vi "Image Display Loop.vi"(0 "fpga interface in":refnum<k20>, 1 "'stop' notifier":refnum<notifier>, 2 "rate references":T1(array[cluster]), 3 "Ctl Refnum":refnum<vi>, 5 "raw display notifier":refnum<notifier>, 7 "display references":refnum<vi>[](array[refnum]), 11 "error in (no error)":errorcluster) -> (15 "error out":errorcluster)   [LabVIEW 2025, in "GettingStarted_Common_148X_Host.lvlib"]
uses:
  GettingStarted_Common_148X_Host.lvlib
  <vilib>/vision/Image Controls.llb/IMAQ Image.ctl
  Types/Serial Channel Display Parameters.ctl
  Types/RAW Interpretation for Display.ctl
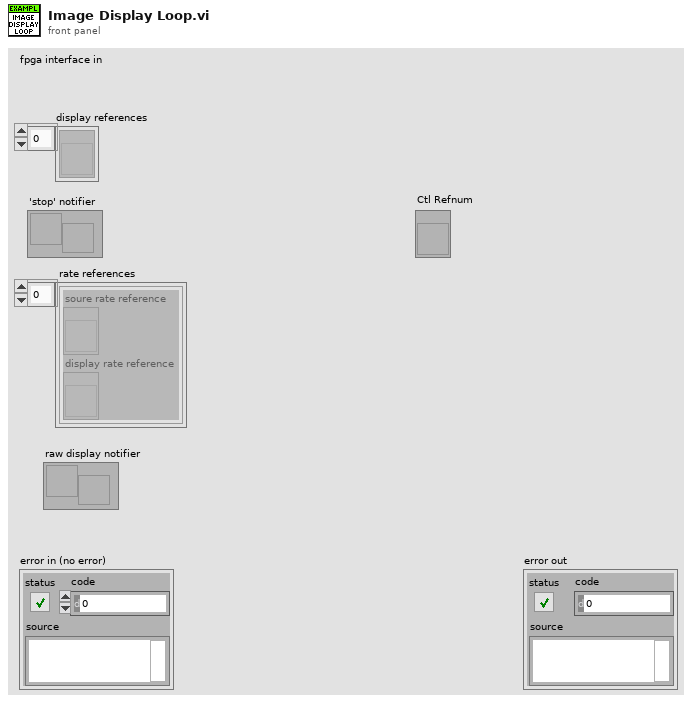
[diagram p1: front panel]
types:
  T1 = cluster{"soure rate reference":refnum<vi>, "display rate reference":refnum<vi>}[]
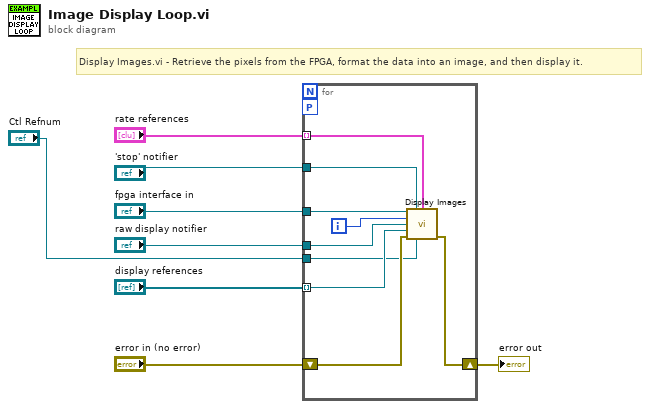
[diagram p0: block diagram]
diagram:
  # "Display Images.vi - Retrieve the pixels from the FPGA, format the data into an image, and then display it."
  n1 = for {
    tunnel: "fpga interface in" -> [w17]
    shift-right: [w14] -> w7
    shift-left: "error in (no error)" -> [w15]
    tunnel: "display references" -> [w16] mode=indexing
    tunnel: "rate references" -> [w12] mode=indexing
    workers-P: _ -> [_]
    tunnel: "'stop' notifier" -> [w11]
    tunnel: "raw display notifier" -> [w10]
    tunnel: "Ctl Refnum" -> [w9]
    i -> [w13]
    n2 = call "Display Images.vi"("fpga interface in"=w17, "'stop' notifier"=w11, "rate references"=w12, "display channel number"=w13, "raw display notifier"=w10, "display reference"=w16, "error in (no error)"=w15, "Ctl Refnum"=w9) -> ("error out"=w14:errorcluster)  [unwired: 6 in, 1 out]
  }
  "error out" <- w7
